vi "Get Audio File Info (Polymorphic Template).vi"   [LabVIEW 2020]
uses:
  4eec47c5-3867-48fc-af9a-773a85a8cbd4.vi
  11be0b8a-0ecf-48c6-ad13-a826563776bf.vi
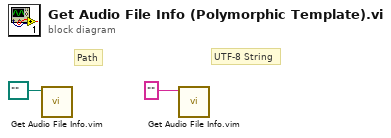
[diagram p0: block diagram]
diagram:
  # "UTF-8 String"
  # "Path"
  n1 = call "Get Audio File Info.vim"("Path In"=path "") -> ()  [unwired: 6 in, 5 out]
  n2 = call "Get Audio File Info.vim"("Path In"="") -> ()  [unwired: 6 in, 5 out]
